vi "odczytywanie.vi"() -> ()   [LabVIEW 2020]
uses:
  <vilib>/Utility/xml.llb/Write to XML File(string).vi
panel:
  out "path":path
  out "natlenienie":dbl(graph)
  out "poziom":dbl(graph)
  in  "Stop Button":bool
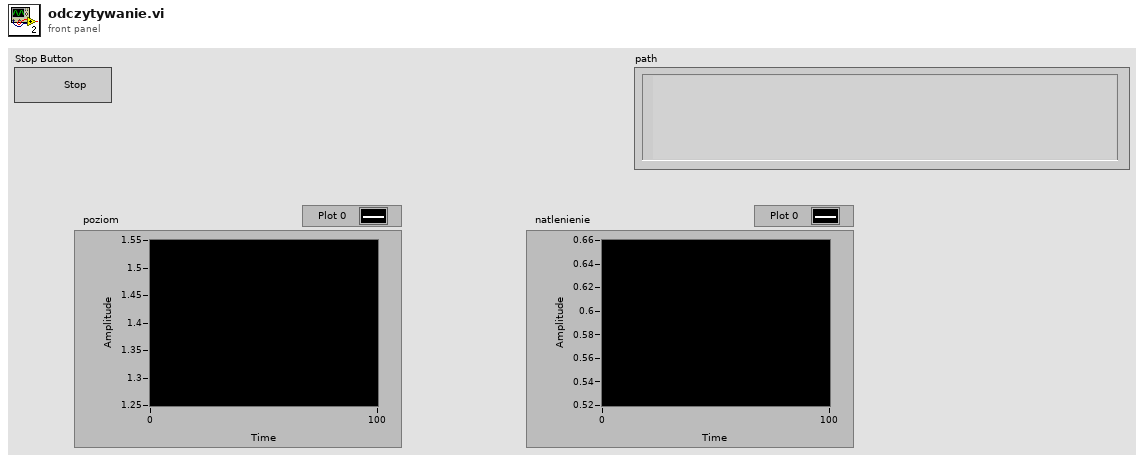
[diagram p1: front panel]
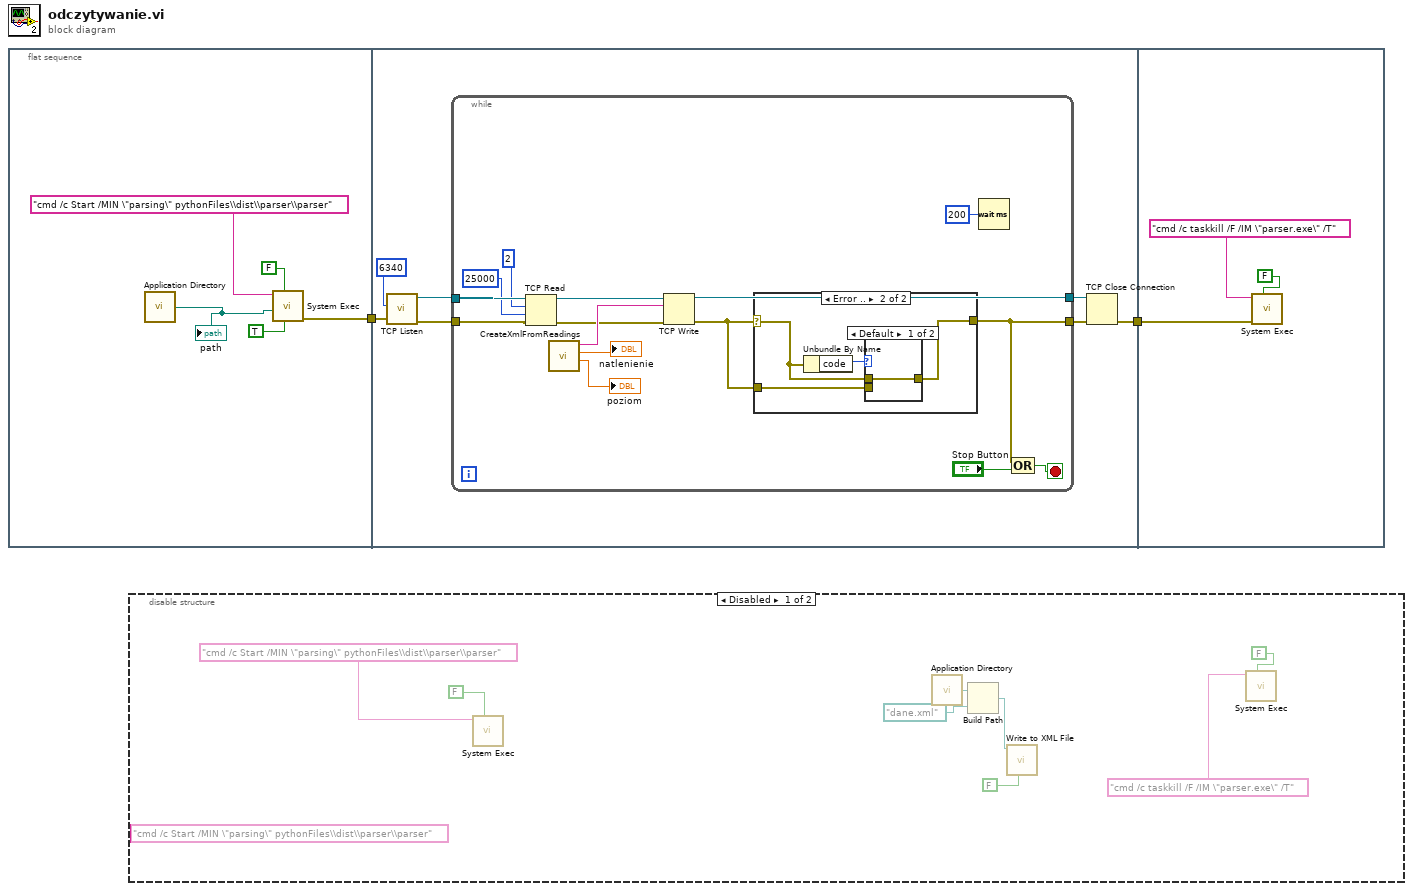
[diagram p0: block diagram]
diagram:
  n1 = flat-sequence {
    tunnel: [w6] -> w2
    tunnel: w2 -> [w11]
    tunnel: [w8] -> w1
    tunnel: w1 -> [w37]
    frame #0 {
      n2 = call <vilib>:"Application Directory.vi"() -> ("Application Directory"=w3:path)
      "path" <- w3
      n3 = call <vilib>:"System Exec.vi"("run minimized? (F)"=TRUE, "wait until completion? (T)"=FALSE, "working directory"=w3, "command line"="cmd /c Start /MIN \"parsing\" pythonFiles\\dist\\parser\\parser") -> ("error out"=w6:errorcluster)  [unwired: 4 in, 3 out]
    }
    frame #1 {
      n4 = call <vilib>:"TCP Listen.vi"("error in (no error)"=w11, "port"=u16 6340) -> ("error out"=w10:errorcluster, "connection ID"=w13:refnum<k5>)  [unwired: 5 in, 3 out]
      n5 = while {
        tunnel: w13 -> [w27]
        tunnel: [w29] -> w12
        tunnel: w10 -> [w20]
        tunnel: [w16] -> w9
        stop <- w17 stop-if-true
        n6 = TCP Read(connection ID=w27, bytes to read=2, error in (no error)=w20, 9:25000 ("timeout ms (25000)")) -> (connection ID out=w26:refnum<k5>, error out=w19:errorcluster)  [unwired: 1 in, 1 out]
        n7 = call "CreateXmlFromReadings.vi"() -> ("poziom"=→"poziom":dbl, "natlenienie"=→"natlenienie":dbl, "xml string"=w21:string)  [unwired: 9 in]
        n8 = TCP Write(connection ID=w26, data in=w21, error in (no error)=w19) -> (connection ID out=w29:refnum<k5>, error out=w15:errorcluster)  [unwired: 1 in, 1 out]
        n9 = case shown="Error .." w15 {
          selector: w15 -> [w30 w32]
          tunnel: [w30 w33] -> w16
          tunnel: w15 -> [_ w31]
          frame No Error {
          }
          frame Error {
            n10 = Unbundle By Name(w32) -> ("code"=w34:i32)
            n11 = case shown="Default" w34 {
              tunnel: w32 -> [w35 _]
              tunnel: w31 -> [_ w36]
              tunnel: [w35 w36] -> w33
              frame Default {
              }
              frame 56 {
              }
            }
          }
        }
        n12 = Wait (ms)(milliseconds to wait=u32 200) -> ()  [unwired: 1 out]
        n13 = Compound Arithmetic op=OR(w16, "Stop Button") -> (w17:bool)
      }
      n14 = TCP Close Connection(connection ID=w12, error in (no error)=w9) -> (error out=w8:errorcluster)  [unwired: 1 in, 1 out]
    }
    frame #2 {
      n15 = call <vilib>:"System Exec.vi"("wait until completion? (T)"=FALSE, "error in (no error)"=w37, "command line"="cmd /c taskkill /F /IM \"parser.exe\" /T") -> ()  [unwired: 5 in, 4 out]
    }
  }
  n16 = disable-structure shown="Disabled" {
    frame Disabled {
      (unwired) "cmd /c Start /MIN \"parsing\" pythonFiles\\dist\\parser\\parser" ("command line")
      n17 = call <vilib>:"System Exec.vi"("wait until completion? (T)"=FALSE, "command line"="cmd /c Start /MIN \"parsing\" pythonFiles\\dist\\parser\\parser") -> ()  [unwired: 6 in, 4 out]
      n18 = call <vilib>:"Application Directory.vi"() -> ("Application Directory"=w46:path)
      n19 = Build Path(base path=w46, name or relative path=path "dane.xml" ("File Path")) -> (appended path=w47:path)
      n20 = call-poly <vilib>:"Write to XML File.vi"("Standalone? (T)"=FALSE, "XML File Path"=w47) -> ()  [unwired: 7 in, 3 out]
      n21 = call <vilib>:"System Exec.vi"("wait until completion? (T)"=FALSE, "command line"="cmd /c taskkill /F /IM \"parser.exe\" /T") -> ()  [unwired: 6 in, 4 out]
    }
    frame Enabled {
    }
  }
